vi "Dictionary to Indicator.vi"(0 "Results (Dictionary)":cluster{"key":string, "value":dbl[]}[](array[cluster]), 5 "AI Channel":i32=1 max=7 step=1, 11 "error in (no error)":errorcluster) -> (4 "X":dbl, 6 "Y":dbl, 8 "R":dbl, 10 "Theta":dbl, 14 "Mean":dbl, 15 "error out":errorcluster)   [LabVIEW 2019, in "Instrument.Lockin.lvlib" / "Instrument UI.Lockin.lvclass"]
uses:
  Instrument UI.Lockin.lvclass
  Instrument.Lockin/Typedefs/Results Type--Enum.ctl
  Instrument.Lockin/Instrument.Lockin.lvclass
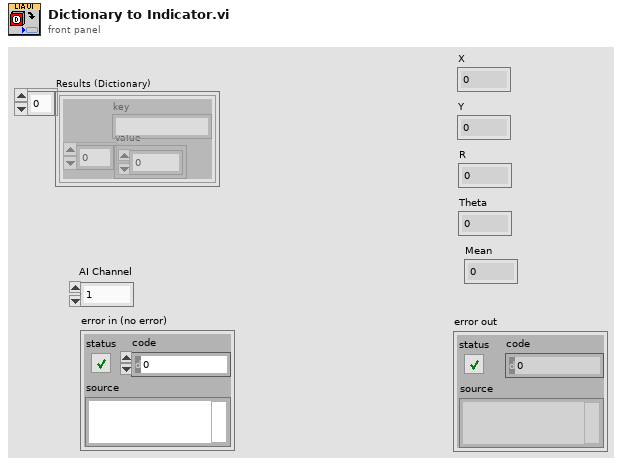
[diagram p1: front panel]
types:
  T1 = typedef "Instrument.Lockin.lvlib/Instrument.Lockin.lvclass/Results Type--Enum.ctl" = enum16{"X", "Y", "R", "Theta", "Mean"}
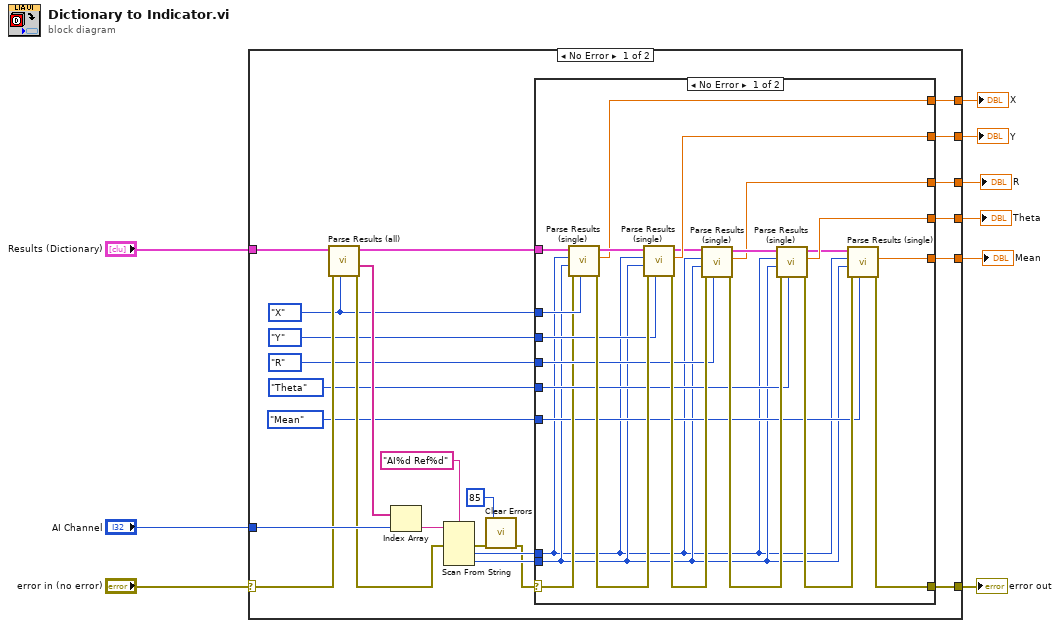
[diagram p0: block diagram]
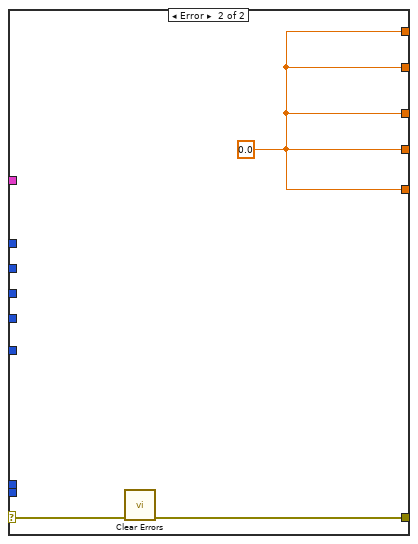
[diagram p2: hidden frame]
diagram:
  n1 = case shown="No Error" "error in (no error)" {
    selector: "error in (no error)" -> [w22 w60]
    tunnel: "Results (Dictionary)" -> [w33 _]
    tunnel: "AI Channel" -> [w29 _]
    tunnel: [w30 _] -> w7
    tunnel: [w31 _] -> w6
    tunnel: [w20 w60] -> w4
    tunnel: [w14 _] -> w2
    tunnel: [w13 _] -> w3
    tunnel: [w10 _] -> w1
    frame No Error {
      w21 = Results_Type--Enum."X" ("Type")
      n2 = call "Parse Results (all).vi"("Type"=w21, "error in (no error)"=w22, "Results (Dictionary)"=w33) -> ("error out"=w27:errorcluster, "Label"=w26:string[], "Results (Dictionary)"=w32:cluster{"key":string, "value":dbl[]}[])  [unwired: 5 in, 1 out]
      n3 = Index Array(array=w26, index=w29) -> (element=w28:string)
      n4 = Scan From String(format string="AI%d Ref%d", input string=w28, error in=w27) -> (error out=w24:errorcluster, output 1=w15:i32, output 2=w16:i32)  [unwired: 3 in, 2 out]
      n5 = call <vilib>:"Clear Errors.vi"("error in (no error)"=w24, "specific error code to clear (0: all)"=85) -> ("error out"=w12:errorcluster)  [unwired: 4 in, 1 out]
      n6 = case shown="No Error" w12 {
        selector: w12 -> [w41 w59]
        tunnel: w32 -> [w56 _]
        tunnel: [w54 w57] -> w31
        tunnel: [w53 w57] -> w30
        tunnel: w21 -> [w51 _]
        tunnel: [w38 w58] -> w20
        tunnel: Results_Type--Enum."Y" ("Type") -> [w47 _]
        tunnel: Results_Type--Enum."R" ("Type") -> [w46 _]
        tunnel: Results_Type--Enum."Theta" ("Type") -> [w44 _]
        tunnel: w16 -> [w36 _]
        tunnel: w15 -> [w35 _]
        tunnel: [w43 w57] -> w14
        tunnel: [w42 w57] -> w13
        tunnel: Results_Type--Enum."Mean" ("Type") -> [w37 _]
        tunnel: [w34 w57] -> w10
        frame No Error {
          n7 = call "Parse Results (single).vi"("Type"=w51, "error in (no error)"=w41, "Reference Channel"=w36, "AI Channel"=w35, "Results (Dictionary)"=w56) -> ("error out"=w52:errorcluster, "Data"=w53:dbl, "Results (Dictionary)"=w55:cluster{"key":string, "value":dbl[]}[])  [unwired: 3 in, 1 out]
          n8 = call "Parse Results (single).vi"("Type"=w47, "error in (no error)"=w52, "Reference Channel"=w36, "AI Channel"=w35, "Results (Dictionary)"=w55) -> ("error out"=w49:errorcluster, "Data"=w54:dbl, "Results (Dictionary)"=w45:cluster{"key":string, "value":dbl[]}[])  [unwired: 3 in, 1 out]
          n9 = call "Parse Results (single).vi"("Type"=w46, "error in (no error)"=w49, "Reference Channel"=w36, "AI Channel"=w35, "Results (Dictionary)"=w45) -> ("error out"=w48:errorcluster, "Data"=w43:dbl, "Results (Dictionary)"=w50:cluster{"key":string, "value":dbl[]}[])  [unwired: 3 in, 1 out]
          n10 = call "Parse Results (single).vi"("Type"=w44, "error in (no error)"=w48, "Reference Channel"=w36, "AI Channel"=w35, "Results (Dictionary)"=w50) -> ("error out"=w39:errorcluster, "Data"=w42:dbl, "Results (Dictionary)"=w40:cluster{"key":string, "value":dbl[]}[])  [unwired: 3 in, 1 out]
          n11 = call "Parse Results (single).vi"("Type"=w37, "error in (no error)"=w39, "Reference Channel"=w36, "AI Channel"=w35, "Results (Dictionary)"=w40) -> ("error out"=w38:errorcluster, "Data"=w34:dbl)  [unwired: 3 in, 2 out]
        }
        frame Error {
          w57 = 0.0 ("Data")
          n12 = call <vilib>:"Clear Errors.vi"("error in (no error)"=w59) -> ("error out"=w58:errorcluster)  [unwired: 5 in, 1 out]
        }
      }
    }
    frame Error {
    }
  }
  "X" <- w7
  "Y" <- w6
  "error out" <- w4
  "R" <- w2
  "Theta" <- w3
  "Mean" <- w1
